vi "NavigateToString.vi"(0 "reference in":refnum<class "DP_WebView.lvclass">, 1 "HTML Content":string, 3 "Timeout(10000ms)":i32=10000, 5 "Error In":errorcluster) -> (14 "reference out":refnum<class "DP_WebView.lvclass">, 15 "Loaded":bool, 19 "Error Out":errorcluster)   [LabVIEW 2020, in "DP_WebView.lvclass"]
doc: "Load dynamic HTML as string"
uses:
  DP_WebView.lvclass
  C:/Projects/DependencyViewer/DependencyViewer/DP_WebView_class/data/Microsoft.Web.WebView2.Core.dll
  data/Microsoft.Web.WebView2.Core.dll
  CallBackVIs/Callback_NavigationComplete.vi
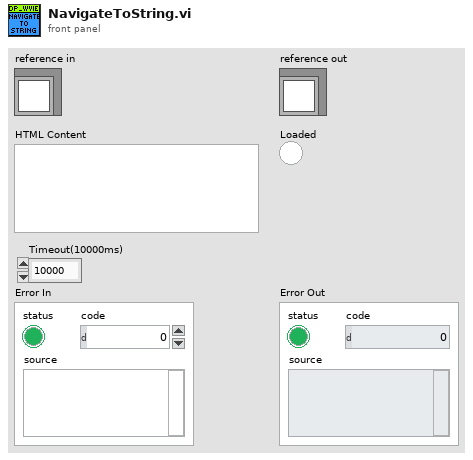
[diagram p1: front panel]
types:
  T1 = typedef "DP_WebView.lvclass/ObjectAttributes.ctl" = cluster{"WebView Container":refnum<k24>, "CoreWebViewRef":refnum<k24>, "Status":i32, "Status Message":string, "User Data Folder":path, "BrowserProcessId":u32}
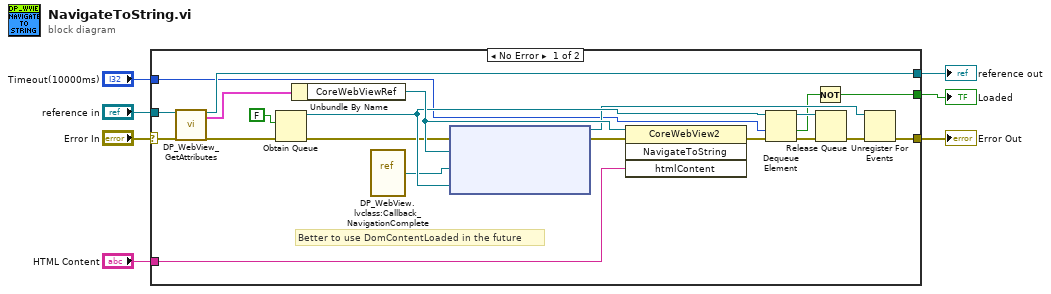
[diagram p0: block diagram]
diagram:
  n1 = case shown="No Error" "Error In" {
    selector: "Error In" -> [w28 w30]
    tunnel: [w10 w30] -> w6
    tunnel: [w26 w29] -> w4
    tunnel: "reference in" -> [w27 w29]
    tunnel: "HTML Content" -> [w11 _]
    tunnel: [w9 _] -> w2
    tunnel: "Timeout(10000ms)" -> [w8 _]
    frame No Error {
      # "Better to use DomContentLoaded in the future"
      n2 = call "DP_WebView_GetAttributes.vi"("reference in"=w27, "error in (no error)"=w28) -> ("reference out"=w26:refnum<class "DP_WebView.lvclass">, "Data"=w13:T1, "error out"=w12:errorcluster)  [unwired: 14 in, 1 out]
      n3 = Obtain Queue(element data type=FALSE ("IsSuccess"), error in (no error)=w12) -> (queue out=w22:refnum<queue>, error out=w21:errorcluster)  [unwired: 3 in, 1 out]
      n4 = Unbundle By Name(w13) -> ("CoreWebViewRef"=w23:refnum<k24>)
      n5 = vi-ref "DP_WebView.lvclass:Callback_NavigationComplete.vi"() -> ("vi reference"=w19:refnum<vi>)
      n6 = node(w21, w23, w19, w22) -> (w20:refnum<k27>, w24:errorcluster)  [unwired: 1 in]
      n7 = invoke class="CoreWebView2" method="NavigateToString"(reference=w23, error in=w24, "htmlContent"=w11) -> (error out=w25:errorcluster)  [unwired: 1 in, 3 out]
      n8 = Dequeue Element(queue=w22, timeout in ms (-1)=w8, error in (no error)=w25) -> (queue out=w17:refnum<queue>, timed out?=w14:bool, error out=w16:errorcluster)  [unwired: 1 out]
      n9 = Not(x=w14) -> (.not. x?=w9:bool)
      n10 = Release Queue(queue=w17, error in (no error)=w16) -> (error out=w15:errorcluster)  [unwired: 1 in, 2 out]
      n11 = Unregister For Events(event registration refnum=w20, error in=w15) -> (error out=w10:errorcluster)
    }
    frame Error {
    }
  }
  "Error Out" <- w6
  "reference out" <- w4
  "Loaded" <- w2
